vi "AOselector.vi"(8 "I/O element":T1(ring), 11 "value":i16) -> ()   [LabVIEW 2023]
uses:
  <vilib>/eio/EIONode/EIONode.xnode
  <vilib>/rvi/eio/common/nirviEmuTemplateMethod_errors.vi
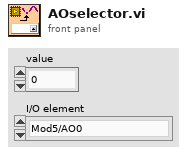
[diagram p1: front panel]
types:
  T1 = enum16{"Mod5/AO0", "Mod5/AO1", "Mod5/AO2", "Mod5/AO3"}
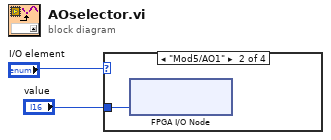
[diagram p0: block diagram]
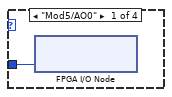
[diagram p2: hidden frame]
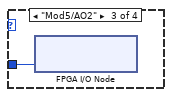
[diagram p3: hidden frame]
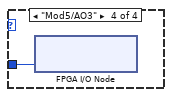
[diagram p4: hidden frame]
diagram:
  n1 = case shown="\"Mod5/AO1\"" "I/O element" {
    tunnel: "value" -> [w3 w4 w5 w6]
    frame "Mod5/AO0" {
      n2 = xnode "FPGA I/O Node"("Mod5/AO0"=w3) -> ()  [unwired: 1 in, 1 out]
    }
    frame "Mod5/AO1" {
      n3 = xnode "FPGA I/O Node"("Mod5/AO1"=w4) -> ()  [unwired: 1 in, 1 out]
    }
    frame "Mod5/AO2" {
      n4 = xnode "FPGA I/O Node"("Mod5/AO2"=w5) -> ()  [unwired: 1 in, 1 out]
    }
    frame "Mod5/AO3" {
      n5 = xnode "FPGA I/O Node"("Mod5/AO3"=w6) -> ()  [unwired: 1 in, 1 out]
    }
  }
